vi "Actor Core.vi"(8 "error in":errorcluster, 11 "MockModel in":refnum<class "TestModelFastPublish.lvclass">) -> (0 "error out":errorcluster, 3 "Actor out":refnum<class "Actor.lvclass">)   [LabVIEW 2017, in "TestModels.lvlib" / "TestModelFastPublish.lvclass"]
doc: "(<B>Filename</B>: Actor Framework.lvlib:Actor.lvclass:Actor Core.vi)\n\nReceives messages to the actor, reacts to them, and initiates any error handling that may shut the actor down.\n\nDescendant classes may override this VI to append parallel tasks for the actor to complete while it handles messages. Overrides use the Call Parent Method node."
uses:
  TestModelFastPublish.lvclass
  C:/Git/mva-framework/Source/Framework/IModel/IModel/IModel.lvclass
  <vilib>/ActorFramework/Actor/Actor.lvclass
  Source/Framework/IObserver/IObserver/IObserver.lvclass/IObserver.ctl
  Source/Framework/IModel/IModel/IModel.lvclass/IModel.ctl
  Source/Framework/IMediator/PublishRequest/PublishRequest.lvclass/PublishRequest.ctl
  Source/Framework/AbstractMessages/PreAddressedMsg/PreAddressedMsg.lvclass/PreAddressedMsg.ctl
  Source/Framework/IMediator/IMediator Messages/Publish Msg/Publish Msg.lvclass/Publish Msg.ctl
  <vilib>/ActorFramework/Message Enqueuer/Message Enqueuer.lvclass/Message Enqueuer.ctl
  Source/Framework/IMediator/IMediator Messages/Publish Msg/Send Pre-Addressed Publish.vi
  Source/Framework/IObserver/IObserver/Read Unique ID.vi
  Source/Framework/IMediator/PublishRequest/Pack Publish Request.vi
  <vilib>/ActorFramework/Message Enqueuer/Enqueue.vi
  Source/Framework/AbstractMessages/PreAddressedMsg/Read Return Address.vi
  Source/Framework/IModel/IModel/IModel.lvclass
  C:/Git/mva-framework/Source/Framework/IObserver/IObserver/IObserver.lvclass
  Source/Framework/IMediator/IMediator Messages/Publish Msg/Publish Msg.lvclass
  C:/Git/mva-framework/Source/Framework/AbstractMessages/PreAddressedMsg/PreAddressedMsg.lvclass
  C:/Program Files (x86)/National Instruments/LabVIEW 2017/vi.lib/ActorFramework/Message/Message.lvclass
  <vilib>/ActorFramework/Message Priority Queue/Priority Enqueue.vi
  Source/Framework/IMediator/PublishRequest/PublishRequest.lvclass
panel:
  in  "Stop Publisher":bool
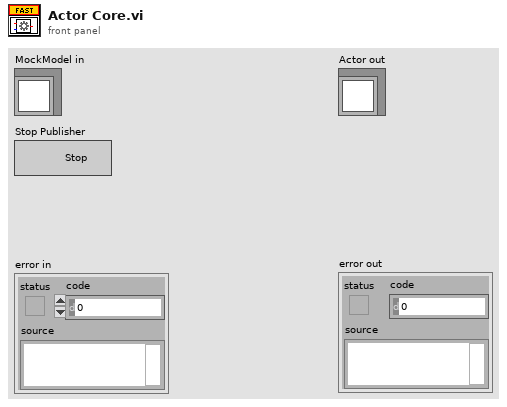
[diagram p1: front panel]
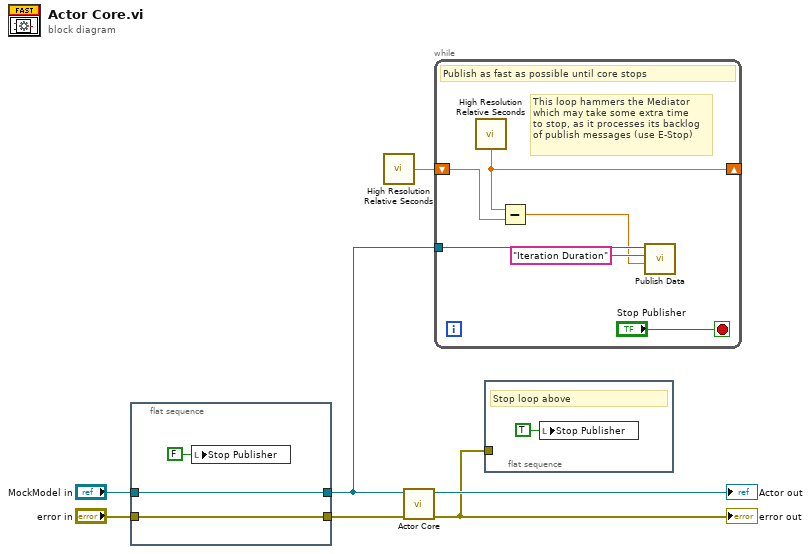
[diagram p0: block diagram]
diagram:
  n1 = flat-sequence {
    tunnel: "error in" -> [w10]
    tunnel: [w10] -> w4
    tunnel: "MockModel in" -> [w9]
    tunnel: [w9] -> w2
    frame #0 {
      n2 = local write "Stop Publisher"(FALSE ("Stop Publisher")) -> ()
    }
  }
  n3 = call <vilib>:"High Resolution Relative Seconds.vi"() -> ("relative seconds"=w1:dbl)
  n4 = call-parent "Actor Core.vi"("error in"=w4, "Actor in"=w2) -> ("error out"=w5:errorcluster, "Actor out"=→"Actor out":refnum<class "Actor.lvclass">)  [unwired: 8 in]
  "error out" <- w5
  n5 = while {
    tunnel: w2 -> [w15]
    shift-right: [w12] -> _
    shift-left: w1 -> [w13]
    stop <- "Stop Publisher" stop-if-true
    # "This loop hammers the Mediator\nwhich may take some extra time\nto stop, as it processes its backlog\nof publish messages (use E-Stop)"
    # "Publish as fast as possible until core stops"
    n6 = call <vilib>:"High Resolution Relative Seconds.vi"() -> ("relative seconds"=w12:dbl)
    n7 = Subtract(x=w12, y=w13) -> (x-y=w11:dbl)
    n8 = call "Publish Data.vi"("Data to Publish"=w11, "Datum Name"="Iteration Duration" ("Topic Name"), "IModel in"=w15) -> ()  [unwired: 7 in, 2 out]
  }
  n9 = flat-sequence {
    tunnel: w5 -> [_]
    frame #0 {
      # "Stop loop above"
      n10 = local write "Stop Publisher"(TRUE ("Stop Publisher")) -> ()
    }
  }
